vi "Adam Asmaca.vi"() -> ()   [LabVIEW 8.6]
uses:
  type_def_Enum_Main_Loop.ctl
panel:
  in  "BASLA":bool
  out "Kelime":string
  in  "Klavye":T1
  out "Adam Asma":T2
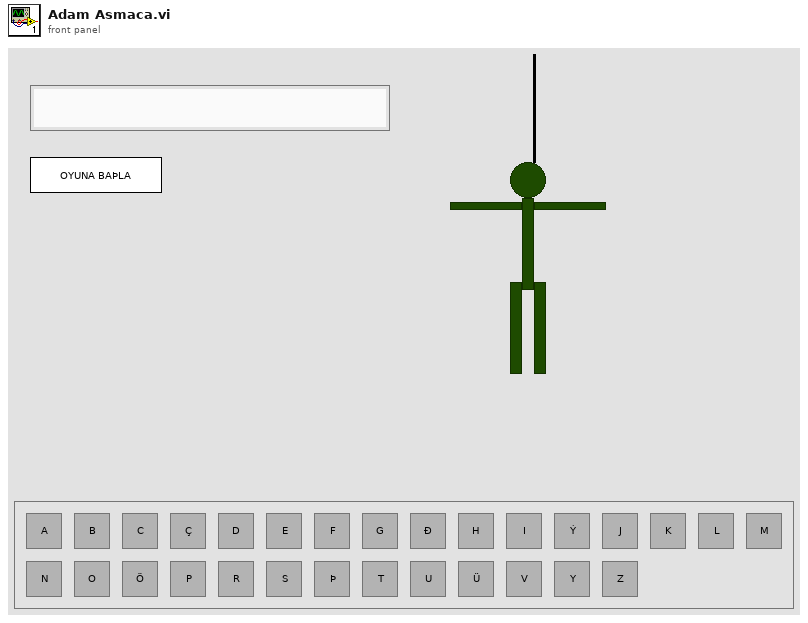
[diagram p1: front panel]
types:
  T1 = cluster{"A":bool, "B":bool, "C":bool, "Ç":bool, "D":bool, "E":bool, "F":bool, "G":bool, "Ð":bool, "H":bool, "I":bool, "Ý":bool, "J":bool, "K":bool, "L":bool, "M":bool, "N":bool, "O":bool, "Ö":bool, "P":bool, "R":bool, "S":bool, "Þ":bool, "T":bool, "U":bool, "Ü":bool, "V":bool, "Y":bool, "Z":bool}
  T2 = cluster{"0":bool, "1":bool, "2":bool, "3":bool, "4":bool, "5":bool}
  T3 = typedef "type_def_Enum_Main_Loop.ctl" = enum16{"Init", "Event", "Start", "Check", "Found", "Not Found", "End"}
  T4 = enum8{"Enabled", "Disabled", "Disabled and Grayed Out"}
  T5 = cluster{"Boolean array[0]":bool, "Boolean array[1]":bool, "Boolean array[2]":bool, "Boolean array[3]":bool, "Boolean array[4]":bool, "Boolean array[5]":bool}
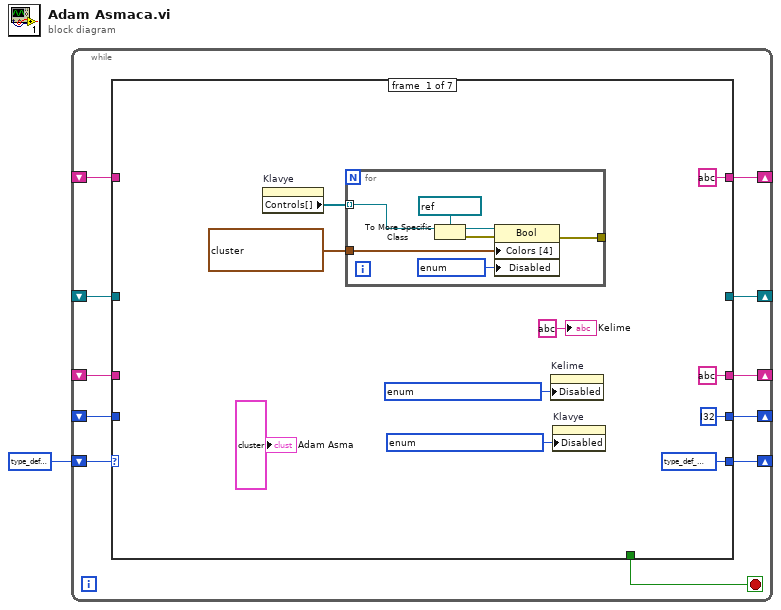
[diagram p0: block diagram]
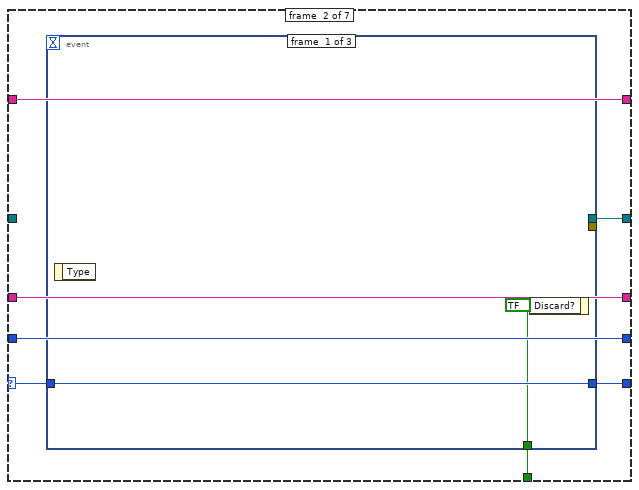
[diagram p2: hidden frame]
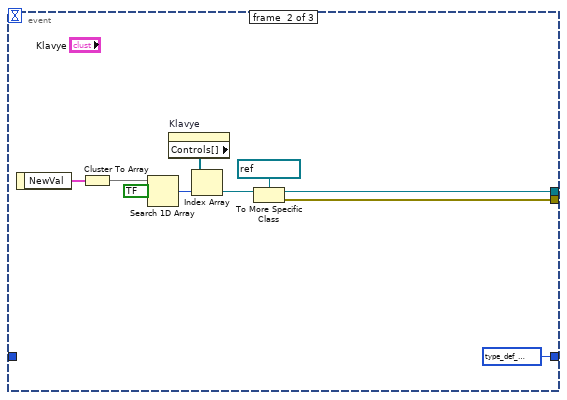
[diagram p3: hidden frame]
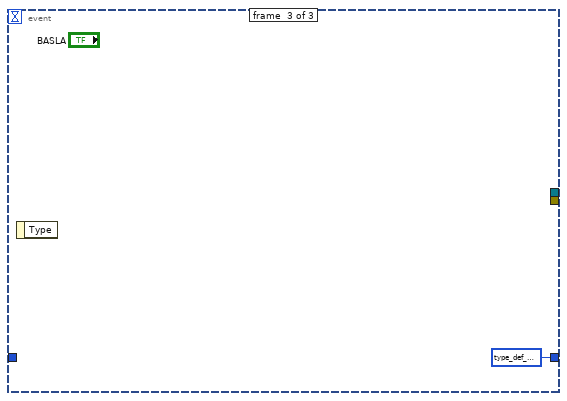
[diagram p4: hidden frame]
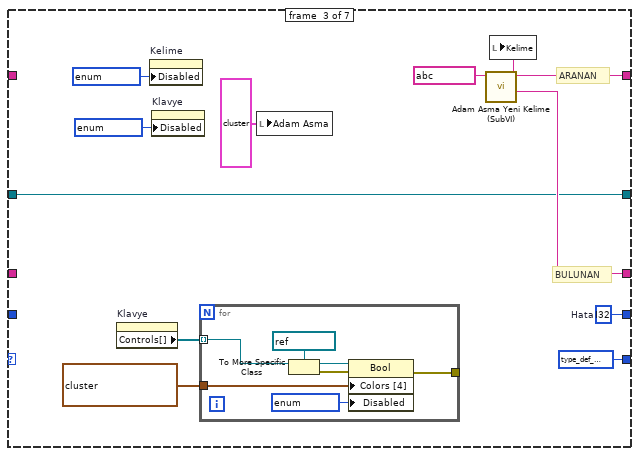
[diagram p5: hidden frame]
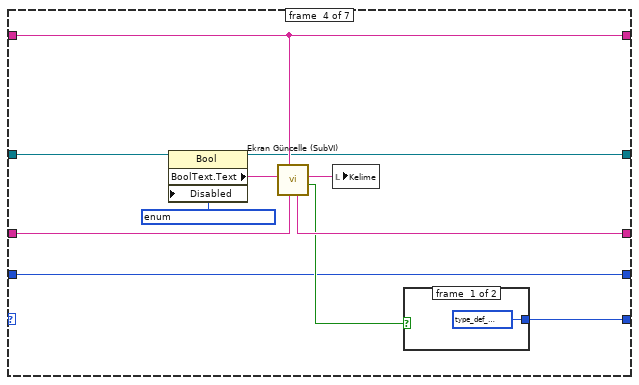
[diagram p6: hidden frame]
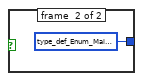
[diagram p7: hidden frame]
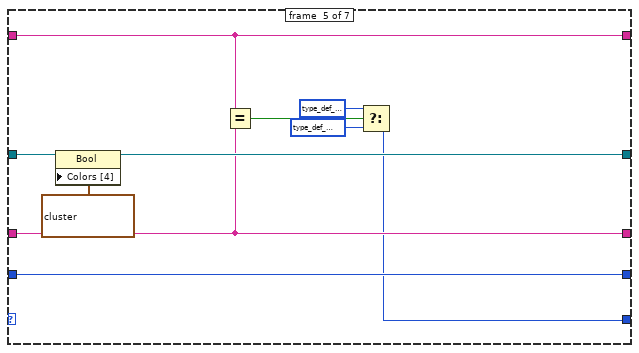
[diagram p8: hidden frame]
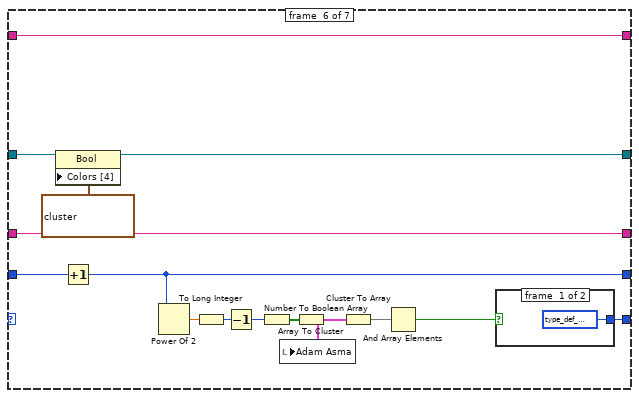
[diagram p9: hidden frame]
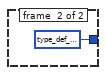
[diagram p10: hidden frame]
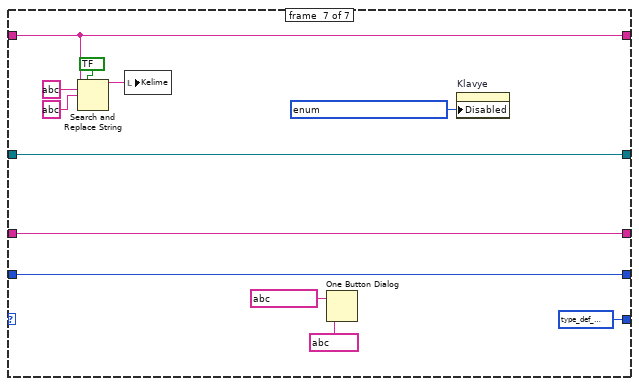
[diagram p11: hidden frame]
diagram:
  n1 = while {
    shift-right: [w12] -> _
    shift-left: _ -> [w11]
    shift-right: [w10] -> _
    shift-left: _ -> [w9]
    shift-right: [w8] -> _
    shift-left: _ -> [w7]
    shift-right: [w5] -> _
    shift-left: T3 ? -> [w6]
    shift-right: [w4] -> _
    shift-left: _ -> [w2]
    stop <- w3 stop-if-true
    n2 = case shown="\"Found\"" w6 {
      selector: w6 -> [_ w34 _ _ _ _ _]
      tunnel: [string ? w33 w59 w77 w87 w106 w112] -> w12
      tunnel: w11 -> [_ w33 _ w77 w87 w106 w112]
      tunnel: [string ? ("Kelime") w32 w58 w79 w86 w105 w119] -> w10
      tunnel: w9 -> [_ w32 _ w78 w86 w105 w119]
      tunnel: [i32 ? ("Bulunan Adet") w36 w57 w71 w91 w95 w118] -> w8
      tunnel: w7 -> [_ w36 _ w71 w91 w104 w118]
      tunnel: [T3 ? w35 T3 ? w70 w82 w103 T3 ?] -> w5
      tunnel: [_ w31 w51 w69 w88 w96 w120] -> w4
      tunnel: [_ w30 _ _ _ _ _] -> w3
      tunnel: w2 -> [_ _ w51 w73 w89 w97 w120]
      frame #0 {
        n3 = property on="Klavye" class="Clust"() -> ("Controls[]"=w15:refnum<vi>[])  [unwired: 2 in, 2 out]
        n4 = for {
          tunnel: w15 -> [w29] mode=indexing
          tunnel: cluster{u32, u32}[] ? ("Colors [4]") -> [w27]
          tunnel: [w26] -> _
          n5 = To More Specific Class(target class=refnum<vi> ? ("Boolean"), reference=w29) -> (specific class reference=w28:refnum<vi>, error out=w23:errorcluster)  [unwired: 1 in]
          n6 = property class="Bool"(reference=w28, error in=w23, "Colors [4]"=w27, "Disabled"=T4 ?) -> (error out=w26:errorcluster)  [unwired: 1 out]
        }
        n7 = property on="Kelime" class="Str"("Disabled"=T4 ?) -> ()  [unwired: 2 in, 2 out]
        n8 = property on="Klavye" class="Clust"("Disabled"=T4 ?) -> ()  [unwired: 2 in, 2 out]
        "Kelime" <- string ? ("Kelime")
        "Adam Asma" <- T2 ? ("Adam Asma")
      }
      frame #1 {
        n9 = event shown="[1] \"Klavye\": Value Change" {
          selector: _ -> [_ _ _]
          dyn-events: _ -> [_ _ _]
          timeout: _ -> [_ _ _]
          tunnel: [w38 T3 ? T3 ?] -> w35
          tunnel: w34 -> [w38 _ _]
          tunnel: [_ w41 _] -> _
          tunnel: [_ w40 _] -> w31
          tunnel: [w37 _ _] -> w30
          event #0 {
            w37 = bool ? ("Discard?")
            n10 = event-data() -> ()  [unwired: 1 in, 1 out]
            n11 = event-data("Discard?"=w37) -> ()  [unwired: 1 in, 1 out]
          }
          event #1 {
            n12 = event-data() -> ("NewVal"=w48:T1)  [unwired: 1 in]
            n13 = Cluster To Array(cluster=w48) -> (array=w47:bool[])
            n14 = Search 1D Array(1D array=w47, element=bool ?) -> (index of element=w44:i32)  [unwired: 1 in]
            n15 = property on="Klavye" class="Clust"() -> ("Controls[]"=w45:refnum<vi>[])  [unwired: 2 in, 2 out]
            n16 = Index Array(array=w45, index=w44) -> (element=w42:refnum<vi>)
            n17 = To More Specific Class(target class=refnum<vi> ? ("Boolean"), reference=w42) -> (specific class reference=w40:refnum<vi>, error out=w41:errorcluster)  [unwired: 1 in]
          }
          event #2 {
            n18 = event-data() -> ()  [unwired: 1 in, 1 out]
          }
        }
      }
      frame #2 {
        w57 = i32 ?  # Hata
        # "BULUNAN"
        # "ARANAN"
        n19 = property on="Klavye" class="Clust"() -> ("Controls[]"=w53:refnum<vi>[])  [unwired: 2 in, 2 out]
        n20 = property on="Kelime" class="Str"("Disabled"=T4 ?) -> ()  [unwired: 2 in, 2 out]
        n21 = property on="Klavye" class="Clust"("Disabled"=T4 ?) -> ()  [unwired: 2 in, 2 out]
        n22 = for {
          tunnel: w53 -> [w68] mode=indexing
          tunnel: cluster{u32, u32}[] ? ("Colors [4]") -> [w66]
          tunnel: [w65] -> _
          n23 = To More Specific Class(target class=refnum<vi> ? ("Boolean"), reference=w68) -> (specific class reference=w67:refnum<vi>, error out=w62:errorcluster)  [unwired: 1 in]
          n24 = property class="Bool"(reference=w67, error in=w62, "Colors [4]"=w66, "Disabled"=T4 ?) -> (error out=w65:errorcluster)  [unwired: 1 out]
        }
        n25 = local write "Adam Asma"(T2 ? ("Adam Asma")) -> ()
        n26 = call "Adam Asma Yeni Kelime (SubVI).vi"("Kelime"=string ?) -> ("Bulunacak"=w58:string, "Görüntülenecek"=w61:string, "Aranacak"=w59:string)  [unwired: 8 in]
        n27 = local write "Kelime"(w61) -> ()
      }
      frame #3 {
        n28 = property class="Bool"(reference=w73, "Disabled"=T4 ?) -> (reference out=w69:refnum<vi>, "BoolText.Text"=w72:string)  [unwired: 1 in, 1 out]
        n29 = call "Ekran Güncelle (SubVI).vi"("Bulunan In"=w78, "Aranan Kelime"=w77, "Harf"=w72) -> ("Bulundu?"=w75:bool, "Görüntü"=w76:string, "Bululnan Out"=w79:string)  [unwired: 6 in]
        n30 = local write "Kelime"(w76) -> ()
        n31 = case shown="False" w75 {
          tunnel: [T3 ? T3 ?] -> w70
          frame #0 {
          }
          frame #1 {
          }
        }
      }
      frame #4 {
        n32 = property class="Bool"(reference=w89, "Colors [4]"=cluster{u32, u32}[] ?) -> (reference out=w88:refnum<vi>)  [unwired: 1 in, 1 out]
        n33 = Equal?(x=w87, y=w86) -> (x = y?=w85:bool)
        n34 = Select(t=T3 ?, s=w85, f=T3 ?) -> (s? t:f=w82:T3)
      }
      frame #5 {
        n35 = property class="Bool"(reference=w97, "Colors [4]"=cluster{u32, u32}[] ?) -> (reference out=w96:refnum<vi>)  [unwired: 1 in, 1 out]
        n36 = Increment(x=w104) -> (x+1=w95:i32)
        n37 = Power Of 2(x=w95) -> (2^x=w101:dbl)
        n38 = To Long Integer(number=w101) -> (32bit integer=w100:i32)
        n39 = Decrement(x=w100) -> (x-1=w99:i32)
        n40 = Number To Boolean Array(number=w99) -> (Boolean array=w102:bool[])
        n41 = Array To Cluster(array=w102) -> (cluster=w94:T5)
        n42 = local write "Adam Asma"(w94) -> ()
        n43 = Cluster To Array(cluster=w94) -> (array=w93:bool[])
        n44 = And Array Elements(Boolean array=w93) -> (logical AND=w92:bool)
        n45 = case shown="True" w92 {
          tunnel: [T3 ? T3 ?] -> w103
          frame #0 {
          }
          frame #1 {
          }
        }
      }
      frame #6 {
        n46 = Search and Replace String(replace all?=bool ? ("replace all? (F)"), input string=w112, search string=string ?, replace string=string ? ("replace string (\"\")")) -> (result string=w116:string)  [unwired: 4 in, 3 out]
        n47 = local write "Kelime"(w116) -> ()
        n48 = One Button Dialog(message=string ?, button name ("OK")=string ?) -> ()  [unwired: 1 out]
        n49 = property on="Klavye" class="Clust"("Disabled"=T4 ?) -> ()  [unwired: 2 in, 2 out]
      }
    }
  }
